vi "AP_2_pulse_control.vi"() -> ()   [LabVIEW 2023]
uses:
  <instrlib>/Quantum Composers 9000 Series/Public/Configure/Configure Chan Mode (Normal).vi
  <instrlib>/Quantum Composers 9000 Series/Quantum Composers 9000 Series.lvlib
panel:
  in  "Gas Pulse Enabled?":bool=TRUE
  in  "Mass Gate Enabled?":bool=TRUE
  in  "Initialization Type":string(combo)="Load from variables "
  in  "Load Conditions":bool
  in  "Save Conditions":bool
  in  "Detachment Laser On?":bool=TRUE
  in  "Detachment Laser Delay / us":dbl=500.0 format="%_4f"
  in  "Laser In Use":string(combo)="QuantaRay 170-30"
  in  "stop":bool
  in  "Mass Gate Width / us":dbl=0.5 format="%_4f"
  in  "Mass Gate Delay / us":dbl=85.0 format="%_4g"
  in  "Repeller Delay / us":dbl=80.0 format="%_4f"
  # "AP2 Delay Controls"
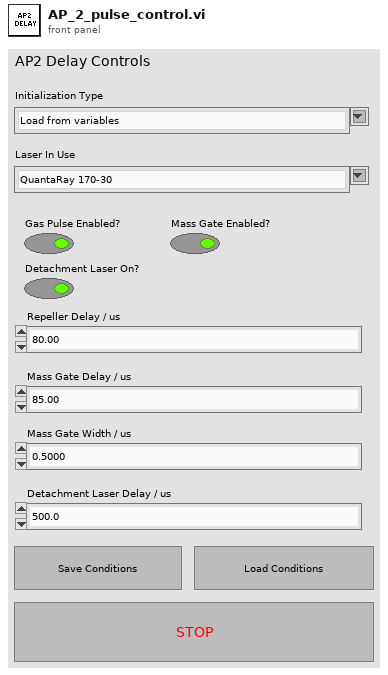
[diagram p1: front panel]
types:
  T1 = cluster{"Mass Gate Delay / us":refnum<vi>, "Mass Gate Width / us":refnum<vi>, "Repeller Delay / us":refnum<vi>, "Mass Gate Enabled?":refnum<vi>, "Gas Pulse Enabled?":refnum<vi>, "Detachment Laser On?":refnum<vi>, "Detachment Laser Delay / us":refnum<vi>}
  T2 = cluster{"Mass Gate Delay / us":dbl, "Mass Gate Width / us":dbl, "Repeller Delay / us":dbl, "Detachment Laser Delay / us":dbl, "Mass Gate Enabled?":bool, "Gas Pulse Enabled?":bool, "Detachment Laser On?":bool}
  T3 = enum16{"Disabled", "Pulse Inhibit", "Output Inhibit"}
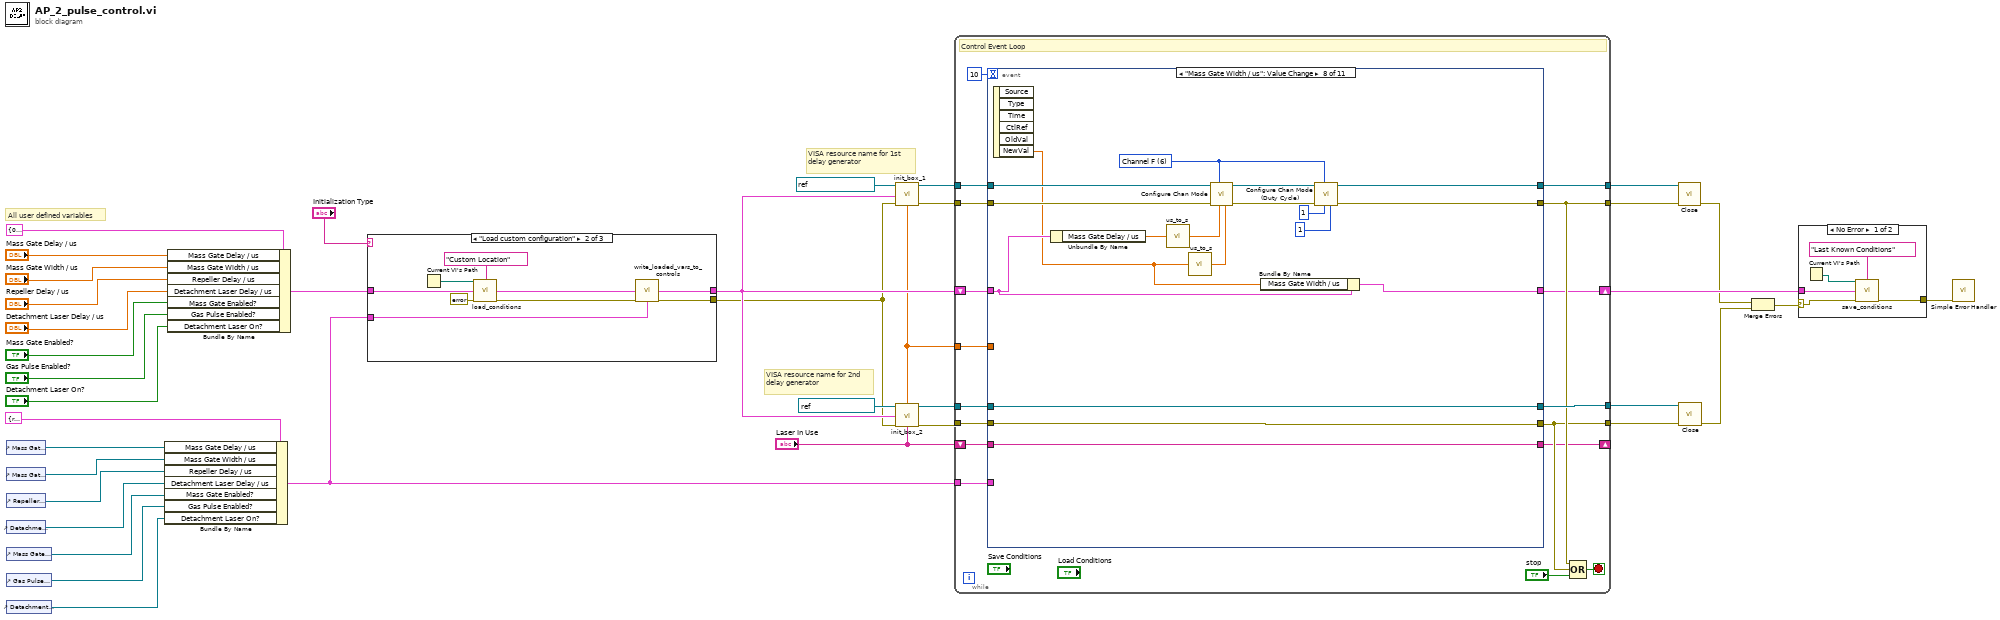
[diagram p0: block diagram]
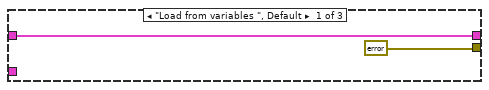
[diagram p2: hidden frame]
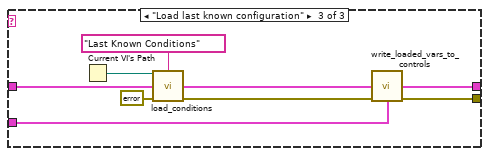
[diagram p3: hidden frame]
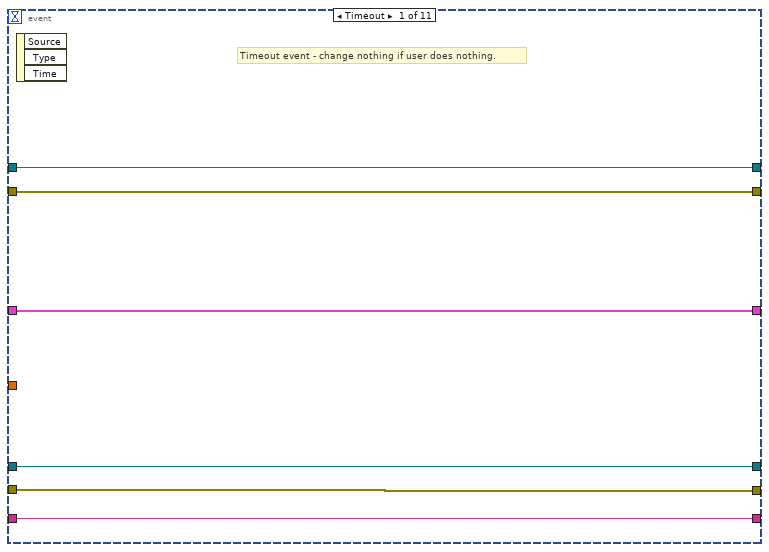
[diagram p5: hidden frame]
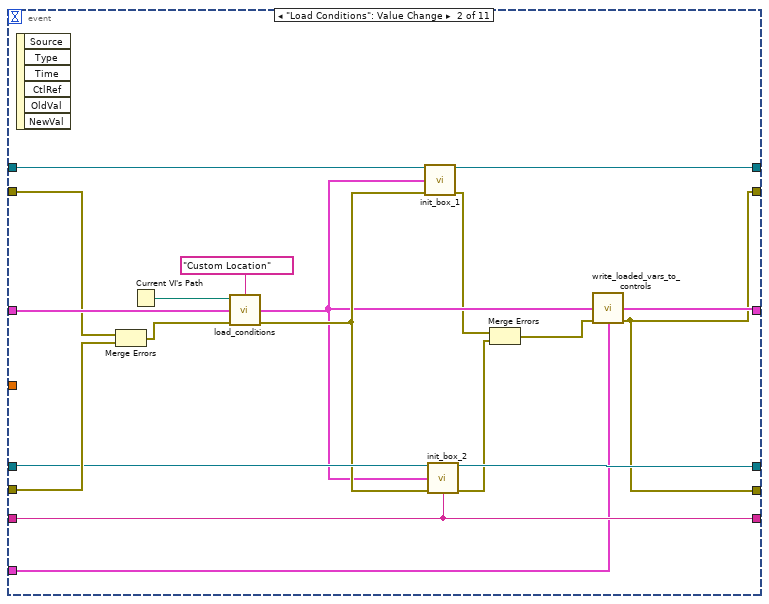
[diagram p6: hidden frame]
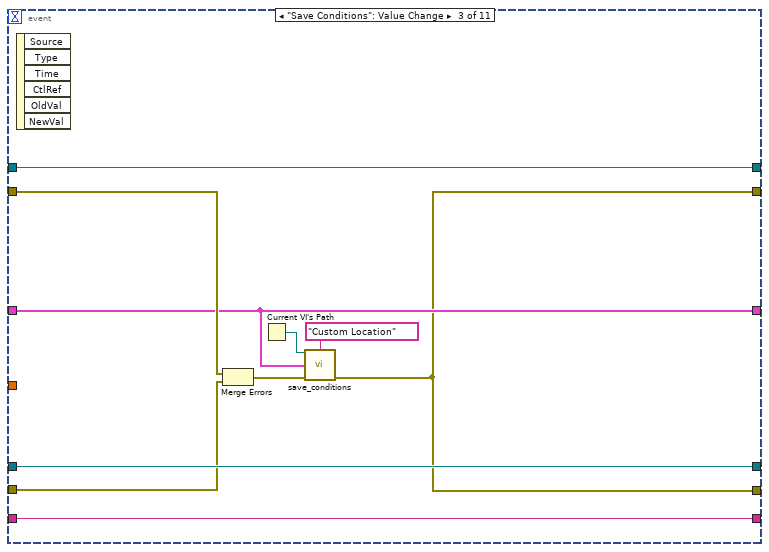
[diagram p7: hidden frame]
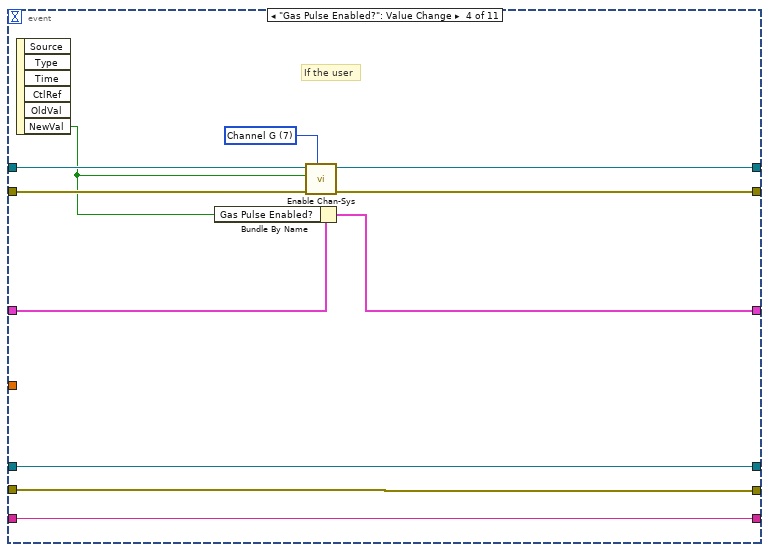
[diagram p8: hidden frame]
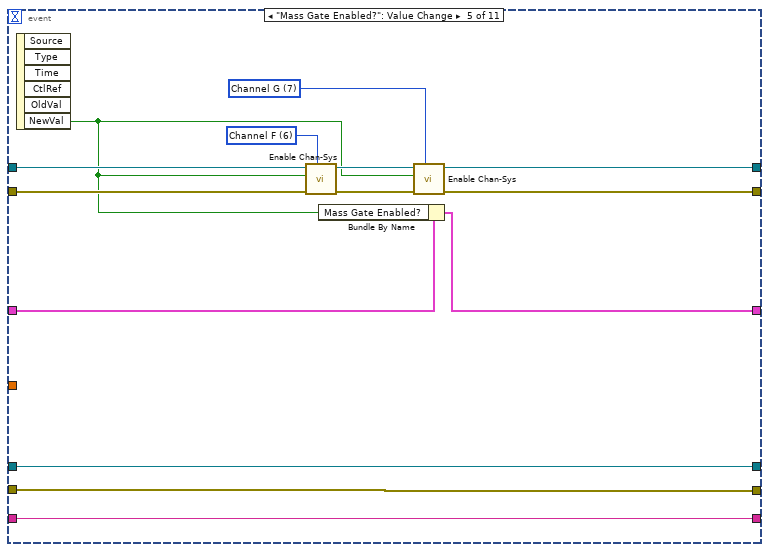
[diagram p9: hidden frame]
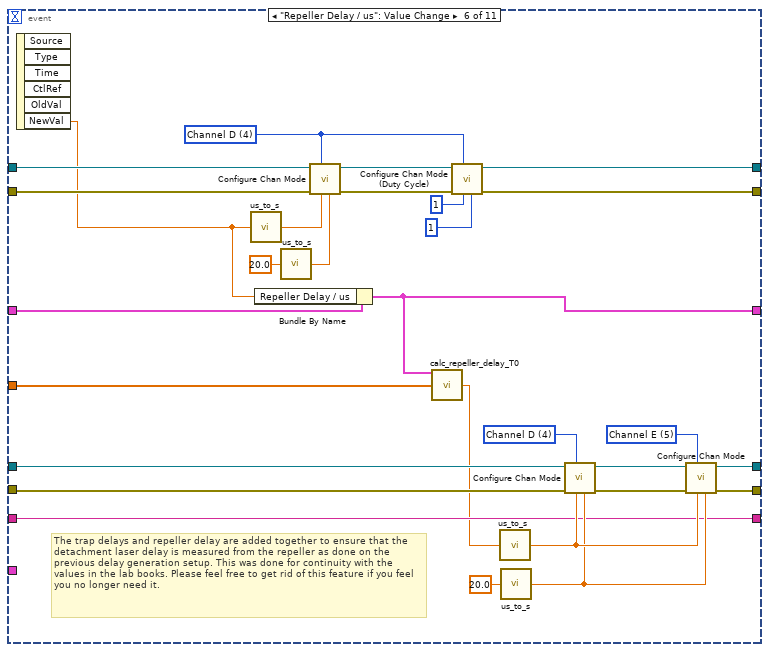
[diagram p10: hidden frame]
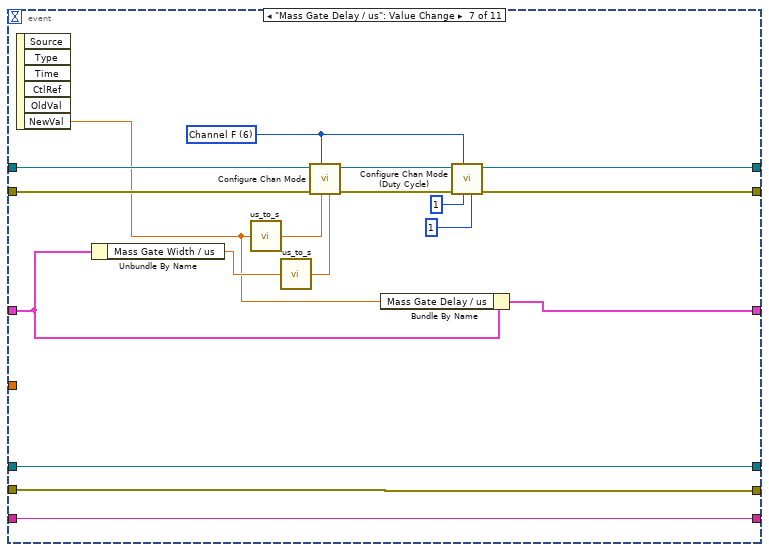
[diagram p11: hidden frame]
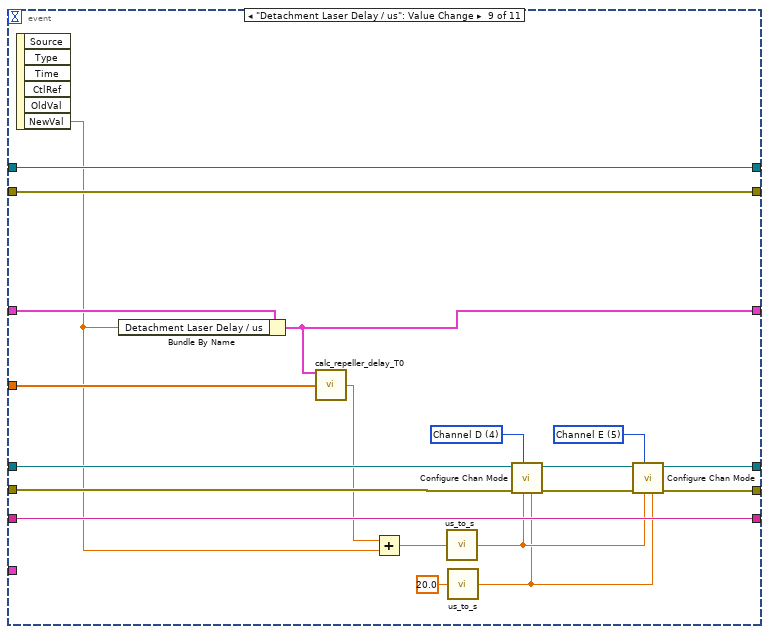
[diagram p12: hidden frame]
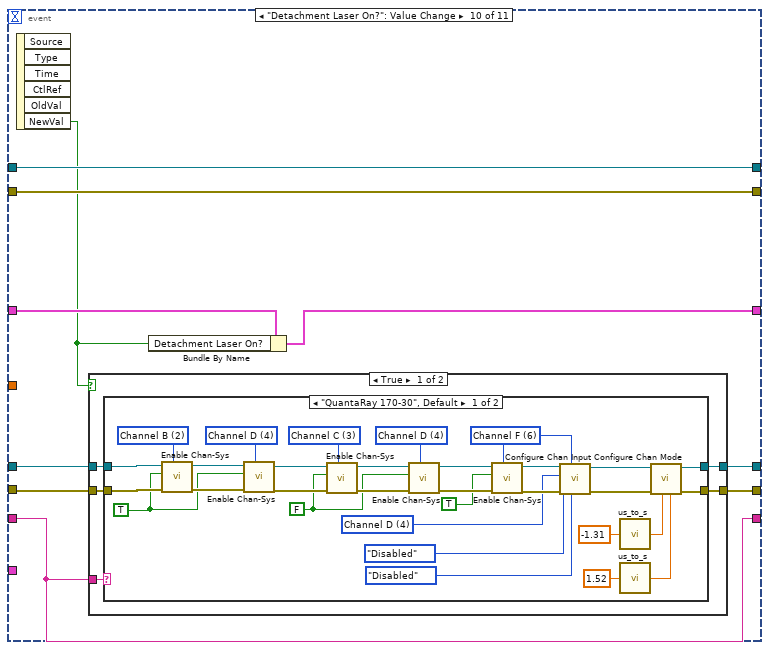
[diagram p13: hidden frame]
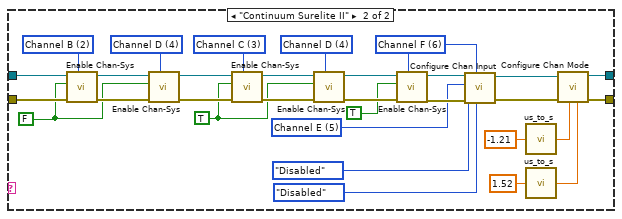
[diagram p14: hidden frame]
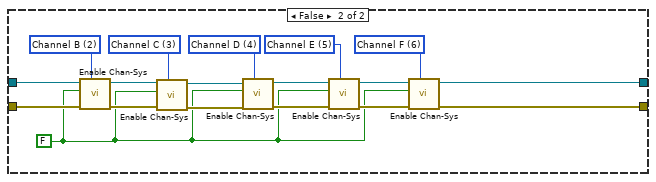
[diagram p15: hidden frame]
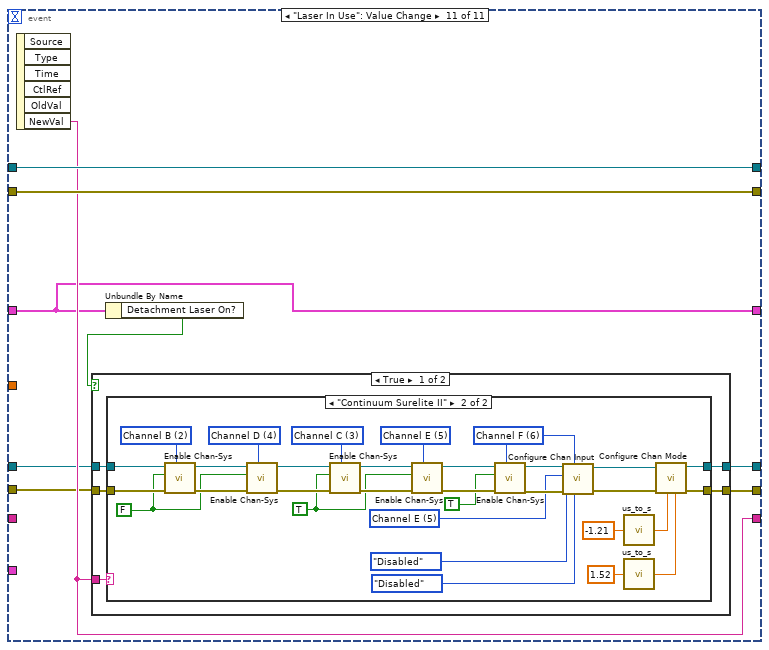
[diagram p16: hidden frame]
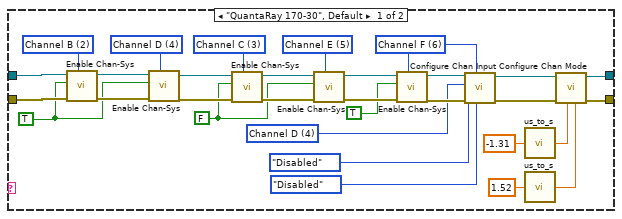
[diagram p17: hidden frame]
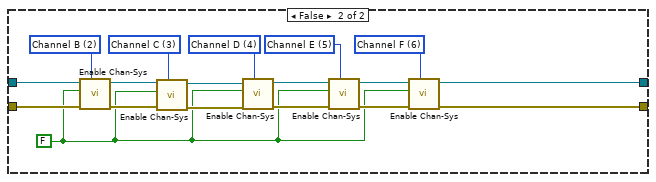
[diagram p18: hidden frame]
diagram:
  # "VISA resource name for 2nd delay generator"
  # "VISA resource name for 1st delay generator"
  # "All user defined variables"
  n1 = control-ref of="Mass Gate Delay / us"() -> (w12:refnum<vi>)
  n2 = control-ref of="Mass Gate Width / us"() -> (w11:refnum<vi>)
  n3 = control-ref of="Repeller Delay / us"() -> (w10:refnum<vi>)
  n4 = control-ref of="Detachment Laser Delay / us"() -> (w9:refnum<vi>)
  n5 = control-ref of="Mass Gate Enabled?"() -> (w2:refnum<vi>)
  n6 = control-ref of="Gas Pulse Enabled?"() -> (w1:refnum<vi>)
  n7 = control-ref of="Detachment Laser On?"() -> (w8:refnum<vi>)
  n8 = Bundle By Name(cluster=T1 {"Mass Gate Delay / us"=refnum, "Mass Gate Width / us"=refnum, "Repeller Delay / us"=refnum, "Mass Gate Enabled?"=refnum, "Gas Pulse Enabled?"=refnum, "Detachment Laser On?"=refnum, "Detachment Laser Delay / us"=refnum}, "Mass Gate Delay / us"=w12, "Mass Gate Width / us"=w11, "Repeller Delay / us"=w10, "Detachment Laser Delay / us"=w9, "Mass Gate Enabled?"=w2, "Gas Pulse Enabled?"=w1, "Detachment Laser On?"=w8) -> (w6:T1)
  n9 = Bundle By Name(cluster=T2 {"Mass Gate Delay / us"=0.0, "Mass Gate Width / us"=0.0, "Repeller Delay / us"=0.0, "Detachment Laser Delay / us"=500.0, "Mass Gate Enabled?"=TRUE, "Gas Pulse Enabled?"=TRUE, "Detachment Laser On?"=FALSE}, "Mass Gate Delay / us"="Mass Gate Delay / us", "Mass Gate Width / us"="Mass Gate Width / us", "Repeller Delay / us"="Repeller Delay / us", "Detachment Laser Delay / us"="Detachment Laser Delay / us", "Mass Gate Enabled?"="Mass Gate Enabled?", "Gas Pulse Enabled?"="Gas Pulse Enabled?", "Detachment Laser On?"="Detachment Laser On?") -> (w16:T2)
  n10 = case shown="\"Load custom configuration\"" "Initialization Type" {
    tunnel: w16 -> [w40 w49 w58]
    tunnel: [w40 w45 w54] -> w15
    tunnel: w6 -> [_ w46 w55]
    tunnel: [errorcluster {"status"=FALSE, "code"=0, "source"=""} ("error in") w43 w52] -> w7
    frame "Load from variables ", Default {
    }
    frame "Load custom configuration" {
      n11 = Current VI's Path() -> (path=w42:path)
      n12 = call "load_conditions.vi"("VI's Path"=w42, "Load Type"="Custom Location", "Config In"=w49, "error in"=errorcluster {"status"=FALSE, "code"=0, "source"=""}) -> ("Config Out"=w48:T2, "error out"=w47:errorcluster)  [unwired: 10 in]
      n13 = call "write_loaded_vars_to_controls.vi"("Variable Values"=w48, "error in (no error)"=w47, "Variable References"=w46) -> ("Variable Values Out"=w45:T2, "error out"=w43:errorcluster)  [unwired: 11 in]
    }
    frame "Load last known configuration" {
      n14 = Current VI's Path() -> (path=w51:path)
      n15 = call "load_conditions.vi"("VI's Path"=w51, "Load Type"="Last Known Conditions", "Config In"=w58, "error in"=errorcluster {"status"=FALSE, "code"=0, "source"=""}) -> ("Config Out"=w57:T2, "error out"=w56:errorcluster)  [unwired: 10 in]
      n16 = call "write_loaded_vars_to_controls.vi"("Variable Values"=w57, "error in (no error)"=w56, "Variable References"=w55) -> ("Variable Values Out"=w54:T2, "error out"=w52:errorcluster)  [unwired: 11 in]
    }
  }
  n17 = call "init_box_1.vi"("Box I VISA Name"=refnum<visa-resource-name> "QC_9530_DG1", "Controls Cluster"=w15, "error in (no error)"=w7) -> ("Box I VISA Name"=w34:refnum<visa-resource-name>, "Trap Delay Array"=w5:dbl[], "error out"=w33:errorcluster)  [unwired: 10 in]
  n18 = call "init_box_2.vi"("Box 2 VISA Name"=refnum<visa-resource-name> "QC_9530_DG2" ("Box I VISA Name"), "Trap Delay Array"=w5, "Controls Cluster"=w15, "error in (no error)"=w7, "Laser In Use"="Laser In Use") -> ("Box 2 VISA Name Out"=w25:refnum<visa-resource-name>, "Error out"=w24:errorcluster)  [unwired: 9 in]
  n19 = while {
    tunnel: w34 -> [w75]
    tunnel: w33 -> [w74]
    tunnel: [w73] -> w38
    tunnel: [w68] -> w37
    tunnel: w25 -> [w71]
    tunnel: w24 -> [w70]
    tunnel: [w69] -> w36
    tunnel: [w67] -> w35
    shift-right: [w63] -> w21
    shift-left: w15 -> [w64]
    shift-right: [w61] -> _
    shift-left: "Laser In Use" -> [w62]
    tunnel: w6 -> [w60]
    tunnel: w5 -> [w59]
    stop <- w66 stop-if-true
    # "Control Event Loop"
    n20 = event shown="[7] \"Mass Gate Width / us\": Value Change" {
      selector: _ -> [_ _ _ _ _ _ _ _ _ _ _]
      dyn-events: _ -> [_ _ _ _ _ _ _ _ _ _ _]
      timeout: 10 -> [_ _ _ _ _ _ _ _ _ _ _]
      tunnel: w75 -> [w81 w99 w110 w118 w132 w164 w180 w198 w220 w230 w324]
      tunnel: w74 -> [w80 w98 w106 w117 w131 w163 w179 w197 w219 w229 w323]
      tunnel: [w81 w91 w110 w116 w125 w137 w176 w194 w220 w230 w324] -> w73
      tunnel: [w80 w84 w101 w115 w124 w136 w175 w193 w219 w229 w323] -> w68
      tunnel: w71 -> [w79 w94 w109 w121 w135 w147 w182 w200 w218 w225 w319]
      tunnel: w70 -> [w78 w97 w107 w120 w134 w146 w181 w199 w217 w224 w318]
      tunnel: [w79 w95 w109 w121 w135 w145 w182 w200 w209 w223 w322] -> w69
      tunnel: [w78 w84 w101 w120 w134 w144 w181 w199 w208 w222 w321] -> w67
      tunnel: w64 -> [w77 w100 w104 w114 w130 w141 w169 w187 w215 w228 w316]
      tunnel: [w77 w90 w104 w113 w129 w139 w168 w186 w204 w227 w316] -> w63
      tunnel: w62 -> [w76 w92 w108 w119 w133 w143 w165 w183 w216 w221 _]
      tunnel: [w76 w92 w108 w119 w133 w143 w165 w183 w216 w221 w320] -> w61
      tunnel: w60 -> [_ w85 _ _ _ _ _ _ _ _ _]
      tunnel: w59 -> [_ _ _ _ _ w142 _ _ w205 _ _]
      event Timeout {
        # "Timeout event - change nothing if user does nothing."
        n21 = event-data() -> ()  [unwired: 1 in, 3 out]
      }
      event "Load Conditions": Value Change {
        n22 = event-data() -> ()  [unwired: 1 in, 6 out]
        n23 = Merge Errors(w98, w97) -> (w96:errorcluster)
        n24 = Current VI's Path() -> (path=w83:path)
        n25 = call "load_conditions.vi"("VI's Path"=w83, "Load Type"="Custom Location", "Config In"=w100, "error in"=w96) -> ("Config Out"=w89:T2, "error out"=w93:errorcluster)  [unwired: 10 in]
        n26 = call "init_box_1.vi"("Box I VISA Name"=w99, "Controls Cluster"=w89, "error in (no error)"=w93) -> ("Box I VISA Name"=w91:refnum<visa-resource-name>, "error out"=w88:errorcluster)  [unwired: 10 in, 1 out]
        n27 = call "init_box_2.vi"("Box 2 VISA Name"=w94, "Controls Cluster"=w89, "error in (no error)"=w93, "Laser In Use"=w92) -> ("Box 2 VISA Name Out"=w95:refnum<visa-resource-name>, "Error out"=w87:errorcluster)  [unwired: 10 in]
        n28 = Merge Errors(w88, w87) -> (w86:errorcluster)
        n29 = call "write_loaded_vars_to_controls.vi"("Variable Values"=w89, "error in (no error)"=w86, "Variable References"=w85) -> ("Variable Values Out"=w90:T2, "error out"=w84:errorcluster)  [unwired: 11 in]
      }
      event "Save Conditions": Value Change {
        n30 = event-data() -> ()  [unwired: 1 in, 6 out]
        n31 = Merge Errors(w106, w107) -> (w105:errorcluster)
        n32 = Current VI's Path() -> (path=w103:path)
        n33 = call "save_conditions.vi"("VI's Path"=w103, "Load Type"="Custom Location" ("Combo Box"), "output cluster"=w104, "error in"=w105) -> ("error out"=w101:errorcluster)  [unwired: 11 in]
      }
      event "Gas Pulse Enabled?": Value Change {
        w111 = 7 items=["System (To)", "Channel A", "Channel B", "Channel C", "Channel D", "Channel E", "Channel F", "Channel G", "Channel H"] ("Channel (1:Chan A)")
        # "If the user"
        n34 = event-data() -> ("NewVal"=w112:bool)  [unwired: 1 in, 5 out]
        n35 = Bundle By Name(cluster=w114, "Gas Pulse Enabled?"=w112) -> (w113:T2)
        n36 = call <instrlib>:"Enable Chan-Sys.vi"("Channel (1:Chan A)"=w111, "error in (no error)"=w117, "State (T:Enabled)"=w112, "VISA resource name"=w118) -> ("error out"=w115:errorcluster, "VISA resource name out"=w116:refnum<visa-resource-name>)  [unwired: 6 in]
      }
      event "Mass Gate Enabled?": Value Change {
        w122 = 7 items=["System (To)", "Channel A", "Channel B", "Channel C", "Channel D", "Channel E", "Channel F", "Channel G", "Channel H"] ("Channel (1:Chan A)")
        w128 = 6 items=["System (To)", "Channel A", "Channel B", "Channel C", "Channel D", "Channel E", "Channel F", "Channel G", "Channel H"] ("Channel (1:Chan A)")
        n37 = event-data() -> ("NewVal"=w123:bool)  [unwired: 1 in, 5 out]
        n38 = call <instrlib>:"Enable Chan-Sys.vi"("Channel (1:Chan A)"=w128, "error in (no error)"=w131, "State (T:Enabled)"=w123, "VISA resource name"=w132) -> ("error out"=w126:errorcluster, "VISA resource name out"=w127:refnum<visa-resource-name>)  [unwired: 6 in]
        n39 = Bundle By Name(cluster=w130, "Mass Gate Enabled?"=w123) -> (w129:T2)
        n40 = call <instrlib>:"Enable Chan-Sys.vi"("Channel (1:Chan A)"=w122, "error in (no error)"=w126, "State (T:Enabled)"=w123, "VISA resource name"=w127) -> ("error out"=w124:errorcluster, "VISA resource name out"=w125:refnum<visa-resource-name>)  [unwired: 6 in]
      }
      event "Repeller Delay / us": Value Change {
        w152 = 5 items=["Channel A"=1, "Channel B"=2, "Channel C"=3, "Channel D"=4, "Channel E"=5, "Channel F"=6, "Channel G"=7, "Channel H"=8] ("Channel (1:Chan A)")
        w153 = 4 items=["Channel A"=1, "Channel B"=2, "Channel C"=3, "Channel D"=4, "Channel E"=5, "Channel F"=6, "Channel G"=7, "Channel H"=8] ("Channel (1:Chan A)")
        w158 = 4 items=["Channel A"=1, "Channel B"=2, "Channel C"=3, "Channel D"=4, "Channel E"=5, "Channel F"=6, "Channel G"=7, "Channel H"=8] ("Channel (1:Chan A)")
        # "The trap delays and repeller delay are added together to ensure that the detachment laser delay is measured from the repeller as done on the previous delay generation setup. This was done for continuity with the values in the lab books. Please feel free to get rid of this feature if you feel you no longer need it."
        n41 = event-data() -> ("NewVal"=w138:dbl)  [unwired: 1 in, 5 out]
        n42 = call "us_to_s.vi"("Time / us"=w138) -> ("Time / s"=w157:dbl)
        n43 = Bundle By Name(cluster=w141, "Repeller Delay / us"=w138) -> (w139:T2)
        n44 = call "us_to_s.vi"("Time / us"=20.0) -> ("Time / s"=w155:dbl)
        n45 = call-poly <instrlib>:"Configure Chan Mode.vi"("Width (10 msec)"=w155, "Delay (10 msec)"=w157, "Channel (1:Chan A)"=w158, "error in (no error)"=w163, "VISA resource name"=w164) -> ("error out"=w161:errorcluster, "VISA resource name out"=w162:refnum<visa-resource-name>)  [unwired: 5 in]
        n46 = call "calc_repeller_delay_T0.vi"("Variable Values Out"=w139, "Trap Delay Array"=w142) -> ("Total Repeller Delay / us"=w140:dbl)  [unwired: 13 in]
        n47 = call <instrlib>:"Configure Chan Mode (Duty Cycle).vi"("Chan DC Off (10)"=1, "Chan DC On (10)"=1, "Channel (1:Chan A)"=w158, "error in (no error)"=w161, "VISA resource name"=w162) -> ("error out"=w136:errorcluster, "VISA resource name out"=w137:refnum<visa-resource-name>)  [unwired: 5 in]
        n48 = call "us_to_s.vi"("Time / us"=w140) -> ("Time / s"=w149:dbl)
        n49 = call "us_to_s.vi"("Time / us"=20.0) -> ("Time / s"=w148:dbl)
        n50 = call-poly <instrlib>:"Configure Chan Mode.vi"("Width (10 msec)"=w148, "Delay (10 msec)"=w149, "Channel (1:Chan A)"=w153, "error in (no error)"=w146, "VISA resource name"=w147) -> ("error out"=w150:errorcluster, "VISA resource name out"=w151:refnum<visa-resource-name>)  [unwired: 5 in]
        n51 = call-poly <instrlib>:"Configure Chan Mode.vi"("Width (10 msec)"=w148, "Delay (10 msec)"=w149, "Channel (1:Chan A)"=w152, "error in (no error)"=w150, "VISA resource name"=w151) -> ("error out"=w144:errorcluster, "VISA resource name out"=w145:refnum<visa-resource-name>)  [unwired: 5 in]
      }
      event "Mass Gate Delay / us": Value Change {
        w172 = 6 items=["Channel A"=1, "Channel B"=2, "Channel C"=3, "Channel D"=4, "Channel E"=5, "Channel F"=6, "Channel G"=7, "Channel H"=8] ("Channel (1:Chan A)")
        n52 = event-data() -> ("NewVal"=w166:dbl)  [unwired: 1 in, 5 out]
        n53 = Unbundle By Name(w169) -> ("Mass Gate Width / us"=w167:dbl)
        n54 = call "us_to_s.vi"("Time / us"=w166) -> ("Time / s"=w171:dbl)
        n55 = call "us_to_s.vi"("Time / us"=w167) -> ("Time / s"=w170:dbl)
        n56 = call-poly <instrlib>:"Configure Chan Mode.vi"("Width (10 msec)"=w170, "Delay (10 msec)"=w171, "Channel (1:Chan A)"=w172, "error in (no error)"=w179, "VISA resource name"=w180) -> ("error out"=w177:errorcluster, "VISA resource name out"=w178:refnum<visa-resource-name>)  [unwired: 5 in]
        n57 = Bundle By Name(cluster=w169, "Mass Gate Delay / us"=w166) -> (w168:T2)
        n58 = call <instrlib>:"Configure Chan Mode (Duty Cycle).vi"("Chan DC Off (10)"=1, "Chan DC On (10)"=1, "Channel (1:Chan A)"=w172, "error in (no error)"=w177, "VISA resource name"=w178) -> ("error out"=w175:errorcluster, "VISA resource name out"=w176:refnum<visa-resource-name>)  [unwired: 5 in]
      }
      event "Mass Gate Width / us": Value Change {
        w190 = 6 items=["Channel A"=1, "Channel B"=2, "Channel C"=3, "Channel D"=4, "Channel E"=5, "Channel F"=6, "Channel G"=7, "Channel H"=8] ("Channel (1:Chan A)")
        n59 = event-data() -> ("NewVal"=w184:dbl)  [unwired: 1 in, 5 out]
        n60 = Unbundle By Name(w187) -> ("Mass Gate Delay / us"=w185:dbl)
        n61 = call "us_to_s.vi"("Time / us"=w185) -> ("Time / s"=w189:dbl)
        n62 = call "us_to_s.vi"("Time / us"=w184) -> ("Time / s"=w188:dbl)
        n63 = call-poly <instrlib>:"Configure Chan Mode.vi"("Width (10 msec)"=w188, "Delay (10 msec)"=w189, "Channel (1:Chan A)"=w190, "error in (no error)"=w197, "VISA resource name"=w198) -> ("error out"=w195:errorcluster, "VISA resource name out"=w196:refnum<visa-resource-name>)  [unwired: 5 in]
        n64 = Bundle By Name(cluster=w187, "Mass Gate Width / us"=w184) -> (w186:T2)
        n65 = call <instrlib>:"Configure Chan Mode (Duty Cycle).vi"("Chan DC Off (10)"=1, "Chan DC On (10)"=1, "Channel (1:Chan A)"=w190, "error in (no error)"=w195, "VISA resource name"=w196) -> ("error out"=w193:errorcluster, "VISA resource name out"=w194:refnum<visa-resource-name>)  [unwired: 5 in]
      }
      event "Detachment Laser Delay / us": Value Change {
        w212 = 5 items=["Channel A"=1, "Channel B"=2, "Channel C"=3, "Channel D"=4, "Channel E"=5, "Channel F"=6, "Channel G"=7, "Channel H"=8] ("Channel (1:Chan A)")
        w213 = 4 items=["Channel A"=1, "Channel B"=2, "Channel C"=3, "Channel D"=4, "Channel E"=5, "Channel F"=6, "Channel G"=7, "Channel H"=8] ("Channel (1:Chan A)")
        n66 = event-data() -> ("NewVal"=w202:dbl)  [unwired: 1 in, 5 out]
        n67 = Bundle By Name(cluster=w215, "Detachment Laser Delay / us"=w202) -> (w204:T2)
        n68 = call "calc_repeller_delay_T0.vi"("Variable Values Out"=w204, "Trap Delay Array"=w205) -> ("Total Repeller Delay / us"=w203:dbl)  [unwired: 13 in]
        n69 = Add(x=w203, y=w202) -> (x+y=w201:dbl)
        n70 = call "us_to_s.vi"("Time / us"=w201) -> ("Time / s"=w207:dbl)
        n71 = call "us_to_s.vi"("Time / us"=20.0) -> ("Time / s"=w206:dbl)
        n72 = call-poly <instrlib>:"Configure Chan Mode.vi"("Width (10 msec)"=w206, "Delay (10 msec)"=w207, "Channel (1:Chan A)"=w213, "error in (no error)"=w217, "VISA resource name"=w218) -> ("error out"=w210:errorcluster, "VISA resource name out"=w211:refnum<visa-resource-name>)  [unwired: 5 in]
        n73 = call-poly <instrlib>:"Configure Chan Mode.vi"("Width (10 msec)"=w206, "Delay (10 msec)"=w207, "Channel (1:Chan A)"=w212, "error in (no error)"=w210, "VISA resource name"=w211) -> ("error out"=w208:errorcluster, "VISA resource name out"=w209:refnum<visa-resource-name>)  [unwired: 5 in]
      }
      event "Detachment Laser On?": Value Change {
        n74 = event-data() -> ("NewVal"=w226:bool)  [unwired: 1 in, 5 out]
        n75 = case shown="True" w226 {
          tunnel: w225 -> [w234 w315]
          tunnel: w224 -> [w233 w314]
          tunnel: [w232 w313] -> w223
          tunnel: [w231 w312] -> w222
          tunnel: w221 -> [w235 _]
          frame True {
            n76 = case shown="\"QuantaRay 170-30\", Default" w235 {
              tunnel: w234 -> [w266 w297]
              tunnel: w233 -> [w265 w296]
              tunnel: [w241 w272] -> w232
              tunnel: [w240 w271] -> w231
              frame "QuantaRay 170-30", Default {
                w245 = FALSE ("State (T:Enabled)")
                w246 = TRUE ("State (T:Enabled)")
                w247 = 4 items=["System (To)", "Channel A", "Channel B", "Channel C", "Channel D", "Channel E", "Channel F", "Channel G", "Channel H"] ("Channel (1:Chan A)")
                w248 = 2 items=["System (To)", "Channel A", "Channel B", "Channel C", "Channel D", "Channel E", "Channel F", "Channel G", "Channel H"] ("Channel (1:Chan A)")
                w249 = 3 items=["System (To)", "Channel A", "Channel B", "Channel C", "Channel D", "Channel E", "Channel F", "Channel G", "Channel H"] ("Channel (1:Chan A)")
                w252 = 4 items=["System (To)", "Channel A", "Channel B", "Channel C", "Channel D", "Channel E", "Channel F", "Channel G", "Channel H"] ("Sync Source (0:To)")
                w256 = 4 items=["System (To)", "Channel A", "Channel B", "Channel C", "Channel D", "Channel E", "Channel F", "Channel G", "Channel H"] ("Channel (1:Chan A)")
                w253 = 6 items=["System (To)", "Channel A", "Channel B", "Channel C", "Channel D", "Channel E", "Channel F", "Channel G", "Channel H"] ("Channel (1:Chan A)")
                n77 = call <instrlib>:"Enable Chan-Sys.vi"("Channel (1:Chan A)"=w248, "error in (no error)"=w265, "State (T:Enabled)"=w246, "VISA resource name"=w266) -> ("error out"=w263:errorcluster, "VISA resource name out"=w264:refnum<visa-resource-name>)  [unwired: 6 in]
                n78 = call <instrlib>:"Enable Chan-Sys.vi"("Channel (1:Chan A)"=w247, "error in (no error)"=w263, "State (T:Enabled)"=w246, "VISA resource name"=w264) -> ("error out"=w261:errorcluster, "VISA resource name out"=w262:refnum<visa-resource-name>)  [unwired: 6 in]
                n79 = call <instrlib>:"Enable Chan-Sys.vi"("Channel (1:Chan A)"=w249, "error in (no error)"=w261, "State (T:Enabled)"=w245, "VISA resource name"=w262) -> ("error out"=w259:errorcluster, "VISA resource name out"=w260:refnum<visa-resource-name>)  [unwired: 6 in]
                n80 = call <instrlib>:"Enable Chan-Sys.vi"("Channel (1:Chan A)"=w256, "error in (no error)"=w259, "State (T:Enabled)"=w245, "VISA resource name"=w260) -> ("error out"=w257:errorcluster, "VISA resource name out"=w258:refnum<visa-resource-name>)  [unwired: 6 in]
                n81 = call <instrlib>:"Enable Chan-Sys.vi"("Channel (1:Chan A)"=w253, "error in (no error)"=w257, "State (T:Enabled)"=TRUE, "VISA resource name"=w258) -> ("error out"=w254:errorcluster, "VISA resource name out"=w255:refnum<visa-resource-name>)  [unwired: 6 in]
                n82 = call <instrlib>:"Configure Chan Input.vi"("Gate Mode (0:Disabled)"=T3."Disabled", "Channel (1:Chan A)"=w253, "error in (no error)"=w254, "Gate Logic (0:Disabled)"=enum16{"Disabled", "Low", "High"}."Disabled", "Sync Source (0:To)"=w252, "VISA resource name"=w255) -> ("error out"=w242:errorcluster, "VISA resource name out"=w243:refnum<visa-resource-name>)  [unwired: 4 in]
                n83 = call "us_to_s.vi"("Time / us"=-1.31) -> ("Time / s"=w237:dbl)
                n84 = call "us_to_s.vi"("Time / us"=1.52) -> ("Time / s"=w236:dbl)
                n85 = call-poly <instrlib>:"Configure Chan Mode.vi"("Width (10 msec)"=w236, "Delay (10 msec)"=w237, "error in (no error)"=w242, "VISA resource name"=w243) -> ("error out"=w240:errorcluster, "VISA resource name out"=w241:refnum<visa-resource-name>)  [unwired: 6 in]
              }
              frame "Continuum Surelite II" {
                w276 = TRUE ("State (T:Enabled)")
                w277 = FALSE ("State (T:Enabled)")
                w278 = 4 items=["System (To)", "Channel A", "Channel B", "Channel C", "Channel D", "Channel E", "Channel F", "Channel G", "Channel H"] ("Channel (1:Chan A)")
                w279 = 2 items=["System (To)", "Channel A", "Channel B", "Channel C", "Channel D", "Channel E", "Channel F", "Channel G", "Channel H"] ("Channel (1:Chan A)")
                w280 = 3 items=["System (To)", "Channel A", "Channel B", "Channel C", "Channel D", "Channel E", "Channel F", "Channel G", "Channel H"] ("Channel (1:Chan A)")
                w283 = 5 items=["System (To)", "Channel A", "Channel B", "Channel C", "Channel D", "Channel E", "Channel F", "Channel G", "Channel H"] ("Sync Source (0:To)")
                w287 = 4 items=["System (To)", "Channel A", "Channel B", "Channel C", "Channel D", "Channel E", "Channel F", "Channel G", "Channel H"] ("Channel (1:Chan A)")
                w284 = 6 items=["System (To)", "Channel A", "Channel B", "Channel C", "Channel D", "Channel E", "Channel F", "Channel G", "Channel H"] ("Channel (1:Chan A)")
                n86 = call <instrlib>:"Enable Chan-Sys.vi"("Channel (1:Chan A)"=w279, "error in (no error)"=w296, "State (T:Enabled)"=w277, "VISA resource name"=w297) -> ("error out"=w294:errorcluster, "VISA resource name out"=w295:refnum<visa-resource-name>)  [unwired: 6 in]
                n87 = call <instrlib>:"Enable Chan-Sys.vi"("Channel (1:Chan A)"=w278, "error in (no error)"=w294, "State (T:Enabled)"=w277, "VISA resource name"=w295) -> ("error out"=w292:errorcluster, "VISA resource name out"=w293:refnum<visa-resource-name>)  [unwired: 6 in]
                n88 = call <instrlib>:"Enable Chan-Sys.vi"("Channel (1:Chan A)"=w280, "error in (no error)"=w292, "State (T:Enabled)"=w276, "VISA resource name"=w293) -> ("error out"=w290:errorcluster, "VISA resource name out"=w291:refnum<visa-resource-name>)  [unwired: 6 in]
                n89 = call <instrlib>:"Enable Chan-Sys.vi"("Channel (1:Chan A)"=w287, "error in (no error)"=w290, "State (T:Enabled)"=w276, "VISA resource name"=w291) -> ("error out"=w288:errorcluster, "VISA resource name out"=w289:refnum<visa-resource-name>)  [unwired: 6 in]
                n90 = call <instrlib>:"Enable Chan-Sys.vi"("Channel (1:Chan A)"=w284, "error in (no error)"=w288, "State (T:Enabled)"=TRUE, "VISA resource name"=w289) -> ("error out"=w285:errorcluster, "VISA resource name out"=w286:refnum<visa-resource-name>)  [unwired: 6 in]
                n91 = call <instrlib>:"Configure Chan Input.vi"("Gate Mode (0:Disabled)"=T3."Disabled", "Channel (1:Chan A)"=w284, "error in (no error)"=w285, "Gate Logic (0:Disabled)"=enum16{"Disabled", "Low", "High"}."Disabled", "Sync Source (0:To)"=w283, "VISA resource name"=w286) -> ("error out"=w273:errorcluster, "VISA resource name out"=w274:refnum<visa-resource-name>)  [unwired: 4 in]
                n92 = call "us_to_s.vi"("Time / us"=-1.21) -> ("Time / s"=w268:dbl)
                n93 = call "us_to_s.vi"("Time / us"=1.52) -> ("Time / s"=w267:dbl)
                n94 = call-poly <instrlib>:"Configure Chan Mode.vi"("Width (10 msec)"=w267, "Delay (10 msec)"=w268, "error in (no error)"=w273, "VISA resource name"=w274) -> ("error out"=w271:errorcluster, "VISA resource name out"=w272:refnum<visa-resource-name>)  [unwired: 6 in]
              }
            }
          }
          frame False {
            w299 = 6 items=["System (To)", "Channel A", "Channel B", "Channel C", "Channel D", "Channel E", "Channel F", "Channel G", "Channel H"] ("Channel (1:Chan A)")
            w300 = 5 items=["System (To)", "Channel A", "Channel B", "Channel C", "Channel D", "Channel E", "Channel F", "Channel G", "Channel H"] ("Channel (1:Chan A)")
            w301 = 4 items=["System (To)", "Channel A", "Channel B", "Channel C", "Channel D", "Channel E", "Channel F", "Channel G", "Channel H"] ("Channel (1:Chan A)")
            w302 = 3 items=["System (To)", "Channel A", "Channel B", "Channel C", "Channel D", "Channel E", "Channel F", "Channel G", "Channel H"] ("Channel (1:Chan A)")
            w298 = FALSE ("State (T:Enabled)")
            w303 = 2 items=["System (To)", "Channel A", "Channel B", "Channel C", "Channel D", "Channel E", "Channel F", "Channel G", "Channel H"] ("Channel (1:Chan A)")
            n95 = call <instrlib>:"Enable Chan-Sys.vi"("Channel (1:Chan A)"=w303, "error in (no error)"=w314, "State (T:Enabled)"=w298, "VISA resource name"=w315) -> ("error out"=w307:errorcluster, "VISA resource name out"=w311:refnum<visa-resource-name>)  [unwired: 6 in]
            n96 = call <instrlib>:"Enable Chan-Sys.vi"("Channel (1:Chan A)"=w302, "error in (no error)"=w307, "State (T:Enabled)"=w298, "VISA resource name"=w311) -> ("error out"=w306:errorcluster, "VISA resource name out"=w310:refnum<visa-resource-name>)  [unwired: 6 in]
            n97 = call <instrlib>:"Enable Chan-Sys.vi"("Channel (1:Chan A)"=w301, "error in (no error)"=w306, "State (T:Enabled)"=w298, "VISA resource name"=w310) -> ("error out"=w305:errorcluster, "VISA resource name out"=w309:refnum<visa-resource-name>)  [unwired: 6 in]
            n98 = call <instrlib>:"Enable Chan-Sys.vi"("Channel (1:Chan A)"=w300, "error in (no error)"=w305, "State (T:Enabled)"=w298, "VISA resource name"=w309) -> ("error out"=w304:errorcluster, "VISA resource name out"=w308:refnum<visa-resource-name>)  [unwired: 6 in]
            n99 = call <instrlib>:"Enable Chan-Sys.vi"("Channel (1:Chan A)"=w299, "error in (no error)"=w304, "State (T:Enabled)"=w298, "VISA resource name"=w308) -> ("error out"=w312:errorcluster, "VISA resource name out"=w313:refnum<visa-resource-name>)  [unwired: 6 in]
          }
        }
        n100 = Bundle By Name(cluster=w228, "Detachment Laser On?"=w226) -> (w227:T2)
      }
      event "Laser In Use": Value Change {
        n101 = event-data() -> ("NewVal"=w320:string)  [unwired: 1 in, 5 out]
        n102 = Unbundle By Name(w316) -> ("Detachment Laser On?"=w317:bool)
        n103 = case shown="True" w317 {
          tunnel: w319 -> [w328 w409]
          tunnel: w318 -> [w327 w408]
          tunnel: [w326 w407] -> w322
          tunnel: [w325 w406] -> w321
          tunnel: w320 -> [w329 _]
          frame True {
            n104 = case shown="\"Continuum Surelite II\"" w329 {
              tunnel: w328 -> [w360 w391]
              tunnel: w327 -> [w359 w390]
              tunnel: [w335 w366] -> w326
              tunnel: [w334 w365] -> w325
              frame "QuantaRay 170-30", Default {
                w339 = FALSE ("State (T:Enabled)")
                w340 = TRUE ("State (T:Enabled)")
                w341 = 4 items=["System (To)", "Channel A", "Channel B", "Channel C", "Channel D", "Channel E", "Channel F", "Channel G", "Channel H"] ("Channel (1:Chan A)")
                w342 = 2 items=["System (To)", "Channel A", "Channel B", "Channel C", "Channel D", "Channel E", "Channel F", "Channel G", "Channel H"] ("Channel (1:Chan A)")
                w343 = 3 items=["System (To)", "Channel A", "Channel B", "Channel C", "Channel D", "Channel E", "Channel F", "Channel G", "Channel H"] ("Channel (1:Chan A)")
                w346 = 4 items=["System (To)", "Channel A", "Channel B", "Channel C", "Channel D", "Channel E", "Channel F", "Channel G", "Channel H"] ("Sync Source (0:To)")
                w350 = 5 items=["System (To)", "Channel A", "Channel B", "Channel C", "Channel D", "Channel E", "Channel F", "Channel G", "Channel H"] ("Channel (1:Chan A)")
                w347 = 6 items=["System (To)", "Channel A", "Channel B", "Channel C", "Channel D", "Channel E", "Channel F", "Channel G", "Channel H"] ("Channel (1:Chan A)")
                n105 = call <instrlib>:"Enable Chan-Sys.vi"("Channel (1:Chan A)"=w342, "error in (no error)"=w359, "State (T:Enabled)"=w340, "VISA resource name"=w360) -> ("error out"=w357:errorcluster, "VISA resource name out"=w358:refnum<visa-resource-name>)  [unwired: 6 in]
                n106 = call <instrlib>:"Enable Chan-Sys.vi"("Channel (1:Chan A)"=w341, "error in (no error)"=w357, "State (T:Enabled)"=w340, "VISA resource name"=w358) -> ("error out"=w355:errorcluster, "VISA resource name out"=w356:refnum<visa-resource-name>)  [unwired: 6 in]
                n107 = call <instrlib>:"Enable Chan-Sys.vi"("Channel (1:Chan A)"=w343, "error in (no error)"=w355, "State (T:Enabled)"=w339, "VISA resource name"=w356) -> ("error out"=w353:errorcluster, "VISA resource name out"=w354:refnum<visa-resource-name>)  [unwired: 6 in]
                n108 = call <instrlib>:"Enable Chan-Sys.vi"("Channel (1:Chan A)"=w350, "error in (no error)"=w353, "State (T:Enabled)"=w339, "VISA resource name"=w354) -> ("error out"=w351:errorcluster, "VISA resource name out"=w352:refnum<visa-resource-name>)  [unwired: 6 in]
                n109 = call <instrlib>:"Enable Chan-Sys.vi"("Channel (1:Chan A)"=w347, "error in (no error)"=w351, "State (T:Enabled)"=TRUE, "VISA resource name"=w352) -> ("error out"=w348:errorcluster, "VISA resource name out"=w349:refnum<visa-resource-name>)  [unwired: 6 in]
                n110 = call <instrlib>:"Configure Chan Input.vi"("Gate Mode (0:Disabled)"=T3."Disabled", "Channel (1:Chan A)"=w347, "error in (no error)"=w348, "Gate Logic (0:Disabled)"=enum16{"Disabled", "Low", "High"}."Disabled", "Sync Source (0:To)"=w346, "VISA resource name"=w349) -> ("error out"=w336:errorcluster, "VISA resource name out"=w337:refnum<visa-resource-name>)  [unwired: 4 in]
                n111 = call "us_to_s.vi"("Time / us"=-1.31) -> ("Time / s"=w331:dbl)
                n112 = call "us_to_s.vi"("Time / us"=1.52) -> ("Time / s"=w330:dbl)
                n113 = call-poly <instrlib>:"Configure Chan Mode.vi"("Width (10 msec)"=w330, "Delay (10 msec)"=w331, "error in (no error)"=w336, "VISA resource name"=w337) -> ("error out"=w334:errorcluster, "VISA resource name out"=w335:refnum<visa-resource-name>)  [unwired: 6 in]
              }
              frame "Continuum Surelite II" {
                w370 = TRUE ("State (T:Enabled)")
                w371 = FALSE ("State (T:Enabled)")
                w372 = 4 items=["System (To)", "Channel A", "Channel B", "Channel C", "Channel D", "Channel E", "Channel F", "Channel G", "Channel H"] ("Channel (1:Chan A)")
                w373 = 2 items=["System (To)", "Channel A", "Channel B", "Channel C", "Channel D", "Channel E", "Channel F", "Channel G", "Channel H"] ("Channel (1:Chan A)")
                w374 = 3 items=["System (To)", "Channel A", "Channel B", "Channel C", "Channel D", "Channel E", "Channel F", "Channel G", "Channel H"] ("Channel (1:Chan A)")
                w377 = 5 items=["System (To)", "Channel A", "Channel B", "Channel C", "Channel D", "Channel E", "Channel F", "Channel G", "Channel H"] ("Sync Source (0:To)")
                w381 = 5 items=["System (To)", "Channel A", "Channel B", "Channel C", "Channel D", "Channel E", "Channel F", "Channel G", "Channel H"] ("Channel (1:Chan A)")
                w378 = 6 items=["System (To)", "Channel A", "Channel B", "Channel C", "Channel D", "Channel E", "Channel F", "Channel G", "Channel H"] ("Channel (1:Chan A)")
                n114 = call <instrlib>:"Enable Chan-Sys.vi"("Channel (1:Chan A)"=w373, "error in (no error)"=w390, "State (T:Enabled)"=w371, "VISA resource name"=w391) -> ("error out"=w388:errorcluster, "VISA resource name out"=w389:refnum<visa-resource-name>)  [unwired: 6 in]
                n115 = call <instrlib>:"Enable Chan-Sys.vi"("Channel (1:Chan A)"=w372, "error in (no error)"=w388, "State (T:Enabled)"=w371, "VISA resource name"=w389) -> ("error out"=w386:errorcluster, "VISA resource name out"=w387:refnum<visa-resource-name>)  [unwired: 6 in]
                n116 = call <instrlib>:"Enable Chan-Sys.vi"("Channel (1:Chan A)"=w374, "error in (no error)"=w386, "State (T:Enabled)"=w370, "VISA resource name"=w387) -> ("error out"=w384:errorcluster, "VISA resource name out"=w385:refnum<visa-resource-name>)  [unwired: 6 in]
                n117 = call <instrlib>:"Enable Chan-Sys.vi"("Channel (1:Chan A)"=w381, "error in (no error)"=w384, "State (T:Enabled)"=w370, "VISA resource name"=w385) -> ("error out"=w382:errorcluster, "VISA resource name out"=w383:refnum<visa-resource-name>)  [unwired: 6 in]
                n118 = call <instrlib>:"Enable Chan-Sys.vi"("Channel (1:Chan A)"=w378, "error in (no error)"=w382, "State (T:Enabled)"=TRUE, "VISA resource name"=w383) -> ("error out"=w379:errorcluster, "VISA resource name out"=w380:refnum<visa-resource-name>)  [unwired: 6 in]
                n119 = call <instrlib>:"Configure Chan Input.vi"("Gate Mode (0:Disabled)"=T3."Disabled", "Channel (1:Chan A)"=w378, "error in (no error)"=w379, "Gate Logic (0:Disabled)"=enum16{"Disabled", "Low", "High"}."Disabled", "Sync Source (0:To)"=w377, "VISA resource name"=w380) -> ("error out"=w367:errorcluster, "VISA resource name out"=w368:refnum<visa-resource-name>)  [unwired: 4 in]
                n120 = call "us_to_s.vi"("Time / us"=-1.21) -> ("Time / s"=w362:dbl)
                n121 = call "us_to_s.vi"("Time / us"=1.52) -> ("Time / s"=w361:dbl)
                n122 = call-poly <instrlib>:"Configure Chan Mode.vi"("Width (10 msec)"=w361, "Delay (10 msec)"=w362, "error in (no error)"=w367, "VISA resource name"=w368) -> ("error out"=w365:errorcluster, "VISA resource name out"=w366:refnum<visa-resource-name>)  [unwired: 6 in]
              }
            }
          }
          frame False {
            w393 = 6 items=["System (To)", "Channel A", "Channel B", "Channel C", "Channel D", "Channel E", "Channel F", "Channel G", "Channel H"] ("Channel (1:Chan A)")
            w394 = 5 items=["System (To)", "Channel A", "Channel B", "Channel C", "Channel D", "Channel E", "Channel F", "Channel G", "Channel H"] ("Channel (1:Chan A)")
            w395 = 4 items=["System (To)", "Channel A", "Channel B", "Channel C", "Channel D", "Channel E", "Channel F", "Channel G", "Channel H"] ("Channel (1:Chan A)")
            w396 = 3 items=["System (To)", "Channel A", "Channel B", "Channel C", "Channel D", "Channel E", "Channel F", "Channel G", "Channel H"] ("Channel (1:Chan A)")
            w392 = FALSE ("State (T:Enabled)")
            w397 = 2 items=["System (To)", "Channel A", "Channel B", "Channel C", "Channel D", "Channel E", "Channel F", "Channel G", "Channel H"] ("Channel (1:Chan A)")
            n123 = call <instrlib>:"Enable Chan-Sys.vi"("Channel (1:Chan A)"=w397, "error in (no error)"=w408, "State (T:Enabled)"=w392, "VISA resource name"=w409) -> ("error out"=w401:errorcluster, "VISA resource name out"=w405:refnum<visa-resource-name>)  [unwired: 6 in]
            n124 = call <instrlib>:"Enable Chan-Sys.vi"("Channel (1:Chan A)"=w396, "error in (no error)"=w401, "State (T:Enabled)"=w392, "VISA resource name"=w405) -> ("error out"=w400:errorcluster, "VISA resource name out"=w404:refnum<visa-resource-name>)  [unwired: 6 in]
            n125 = call <instrlib>:"Enable Chan-Sys.vi"("Channel (1:Chan A)"=w395, "error in (no error)"=w400, "State (T:Enabled)"=w392, "VISA resource name"=w404) -> ("error out"=w399:errorcluster, "VISA resource name out"=w403:refnum<visa-resource-name>)  [unwired: 6 in]
            n126 = call <instrlib>:"Enable Chan-Sys.vi"("Channel (1:Chan A)"=w394, "error in (no error)"=w399, "State (T:Enabled)"=w392, "VISA resource name"=w403) -> ("error out"=w398:errorcluster, "VISA resource name out"=w402:refnum<visa-resource-name>)  [unwired: 6 in]
            n127 = call <instrlib>:"Enable Chan-Sys.vi"("Channel (1:Chan A)"=w393, "error in (no error)"=w398, "State (T:Enabled)"=w392, "VISA resource name"=w402) -> ("error out"=w406:errorcluster, "VISA resource name out"=w407:refnum<visa-resource-name>)  [unwired: 6 in]
          }
        }
      }
    }
    n128 = Compound Arithmetic op=OR(w68, w67, "stop") -> (w66:bool)
  }
  n129 = call <instrlib>:"Close.vi"("error in (no error)"=w37, "VISA resource name"=w38) -> ("error out"=w19:errorcluster)  [unwired: 9 in]
  n130 = call <instrlib>:"Close.vi"("error in (no error)"=w35, "VISA resource name"=w36) -> ("error out"=w20:errorcluster)  [unwired: 9 in]
  n131 = Merge Errors(w19, w20) -> (w17:errorcluster)
  n132 = case shown="No Error" w17 {
    selector: w17 -> [w410 w415]
    tunnel: w21 -> [w414 _]
    tunnel: [w411 w415] -> w18
    frame No Error {
      n133 = Current VI's Path() -> (path=w413:path)
      n134 = call "save_conditions.vi"("VI's Path"=w413, "Load Type"="Last Known Conditions" ("Combo Box"), "output cluster"=w414, "error in"=w410) -> ("error out"=w411:errorcluster)  [unwired: 11 in]
    }
    frame Error {
    }
  }
  n135 = call <vilib>:"Simple Error Handler.vi"("error in (no error)"=w18) -> ()  [unwired: 4 in, 5 out]
